vi "Query Output.vi"(8 "error in":errorcluster, 11 "6509 in":refnum<class "6509.lvclass">) -> (0 "error out":errorcluster, 2 "Port Array":u8[](array[numeric]), 3 "6509 out":refnum<class "6509.lvclass">)   [LabVIEW 2019, in "6509.lvlib" / "6509.lvclass"]
doc: "This method must be overridden by the child class.\n\nThis should read the status at the output of the device and return a weform capture of the named signal states."
uses:
  Library/6509.lvclass
  Library/6509.lvclass/6509.ctl
  <vilib>/DAQmx/read.llb/DAQmx Read (Digital 1D U8 NChan 1Samp).vi
  <vilib>/DAQmx/miscellaneous.llb/DAQmx Fill In Error Info.vi
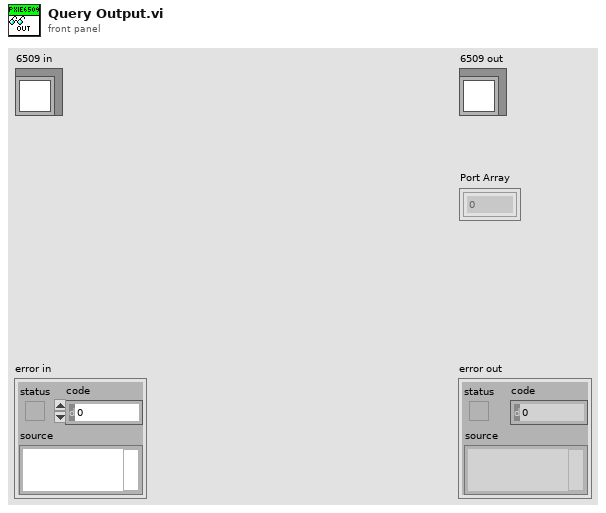
[diagram p1: front panel]
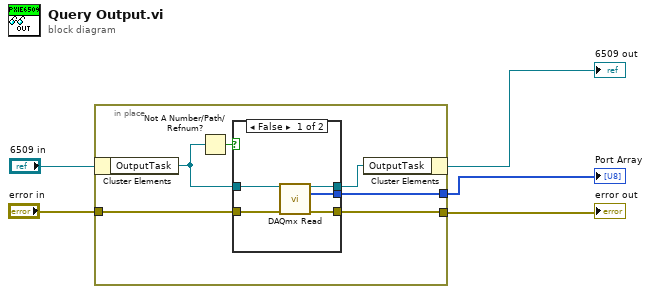
[diagram p0: block diagram]
diagram:
  n1 = in-place {
    in-place-border: [w11] -> w5
    in-place-border: "error in" -> [w9]
    in-place-border: [w8] -> w1
    n2 = in-place-cluster #1("6509 in") -> ("OutputTask"=w7:refnum<k21>)
    n3 = Not A Number/Path/Refnum?(number/path/refnum=w7) -> (NaN/Path/Refnum?=w6:bool)
    n4 = case shown="False" w6 {
      tunnel: [w16 _] -> w11
      tunnel: [w15 w18] -> w10
      tunnel: w9 -> [w14 w17]
      tunnel: [w13 w17] -> w8
      tunnel: w7 -> [w12 w18]
      frame False {
        n5 = call-poly <vilib>:"DAQmx Read.vi"("task/channels in"=w12, "error in"=w14) -> ("task out"=w15:refnum<k21>, "data"=w16:u8[], "error out"=w13:errorcluster)  [unwired: 11 in]
      }
      frame True {
      }
    }
    n6 = in-place-cluster #1("OutputTask"=w10) -> (→"6509 out":refnum<class "6509.lvclass">)
  }
  "error out" <- w1
  "Port Array" <- w5
